vi "Case Structure 2.vi"() -> ()   [LabVIEW 2020]
panel:
  in  "stop":bool
  in  "Play a Sound":bool
  in  "Say Something":bool
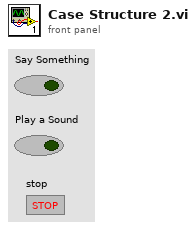
[diagram p1: front panel]
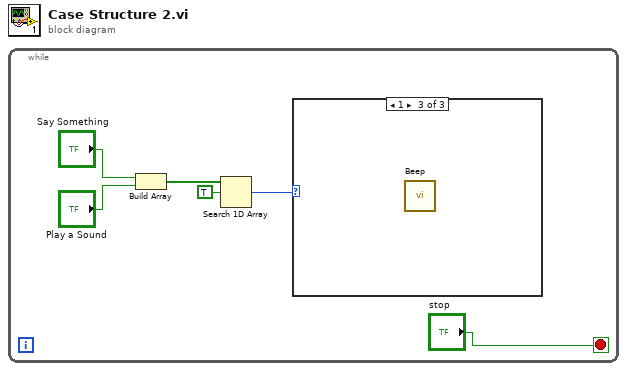
[diagram p0: block diagram]
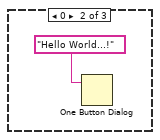
[diagram p3: hidden frame]
diagram:
  n1 = while {
    stop <- "stop" stop-if-true
    n2 = Build Array "Build Array"("Say Something", "Play a Sound") -> (w4:bool[])
    n3 = Search 1D Array(1D array=w4, element=TRUE) -> (index of element=w2:i32)  [unwired: 1 in]
    n4 = case shown="1" w2 {
      frame -1, Default {
      }
      frame 0 {
        n5 = One Button Dialog(message="Hello World...!") -> ()  [unwired: 1 in, 1 out]
      }
      frame 1 {
        n6 = call <vilib>:"Beep.vi"() -> ()  [unwired: 12 in]
      }
    }
  }
